vi "Intake_Globals.vi"() -> ()   [LabVIEW 2019]
uses:
  Intake_States.ctl
  Intake_Cluster.ctl
panel:
  out "Intake_Running":bool
  out "Intake_Extended":bool
  in  "Intake_Left":string
  in  "Intake_Set_Notifier":refnum<notifier>
  in  "Intake_Execute_Notifier":refnum<notifier>
  in  "Intake_Right":string
  in  "Intake_Execute_Ref":string
  in  "Intake_Set_Ref":string
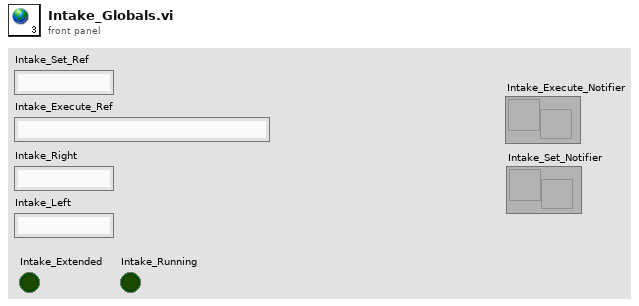
[diagram p1: front panel]
diagram:
